vi "Event Handler.vi"(8 "error in (no error)":errorcluster, 10 "Stop Event Handler":refnum<user-event>, 11 "Cleaningcycle in":refnum<class "Cleaning cycle.lvclass">) -> (0 "error out":errorcluster)   [LabVIEW 2022 SP3, in "Cleaning cycle.lvclass"]
doc: "The <b>Event Handler VI</b> is a dynamic dispatch VI that should be overwritten if events are needed to create the enhanced QControl. \n\nBy inheriting from the main Control.lvclass the overwritten <b>Event Handler VI</b> will be launched asynchronously in the initialization of the QControl.\n<b> </b> <b> </b>\n©2016 Q Software Innovations, LLC (QSI)\nwritten by Quentin Alldredge\nproduced in LabVIEW 2015\n\nsupport@qsoftwareinnovations.com\nwww.qsoftwareinnovations.com\n\nAll rights reserved.\n\nRedistribution and use in source and binary forms, with or without modification, are permitted provided that the following conditions are met:\n\n * Redistributions of source code must retain the above copyright notice, this list of conditions and the following disclaimer.\n * Redistributions in binary form must reproduce the above copyright notice, this list of conditions and the following disclaimer in the documentation and/or other materials provided with the distribution.\n * Neither the name of Q Software Innovations, LLC. nor the names of its contributors may be used to endorse or promote products derived from this software without specific prior written permission.\n\nTHIS SOFTWARE IS PROVIDED BY THE COPYRIGHT HOLDERS AND CONTRIBUTORS \"AS IS\" AND ANY EXPRESS OR IMPLIED WARRANTIES, INCLUDING, BUT NOT LIMITED TO, THE IMPLIED WARRANTIES OF MERCHANTABILITY AND FITNESS FOR A PARTICULAR PURPOSE ARE DISCLAIMED. IN NO EVENT SHALL THE COPYRIGHT OWNER OR CONTRIBUTORS BE LIABLE FOR ANY DIRECT, INDIRECT, INCIDENTAL, SPECIAL, EXEMPLARY, OR CONSEQUENTIAL DAMAGES (INCLUDING, BUT NOT LIMITED TO, PROCUREMENT OF SUBSTITUTE GOODS OR SERVICES; LOSS OF USE, DATA, OR PROFITS; OR BUSINESS INTERRUPTION) HOWEVER CAUSED AND ON ANY THEORY OF LIABILITY, WHETHER IN CONTRACT, STRICT LIABILITY, OR TORT (INCLUDING NEGLIGENCE OR OTHERWISE) ARISING IN ANY WAY OUT OF THE USE OF THIS SOFTWARE, EVEN IF ADVISED OF THE POSSIBILITY OF SUCH DAMAGE."
uses:
  Cleaning cycle.lvclass
  Cleaning cycle.lvclass/Cleaning cycle.ctl
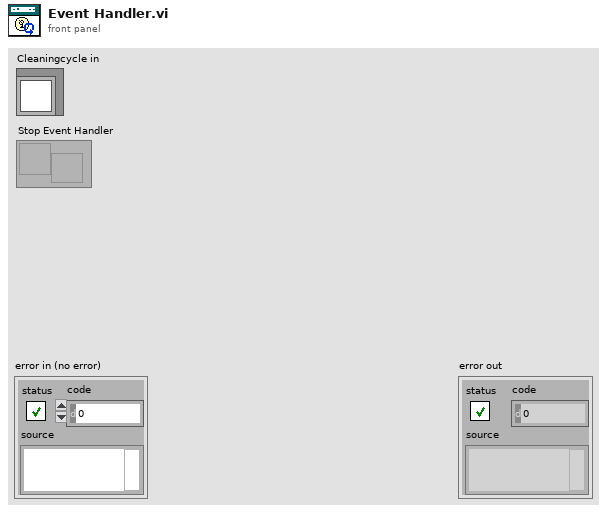
[diagram p1: front panel]
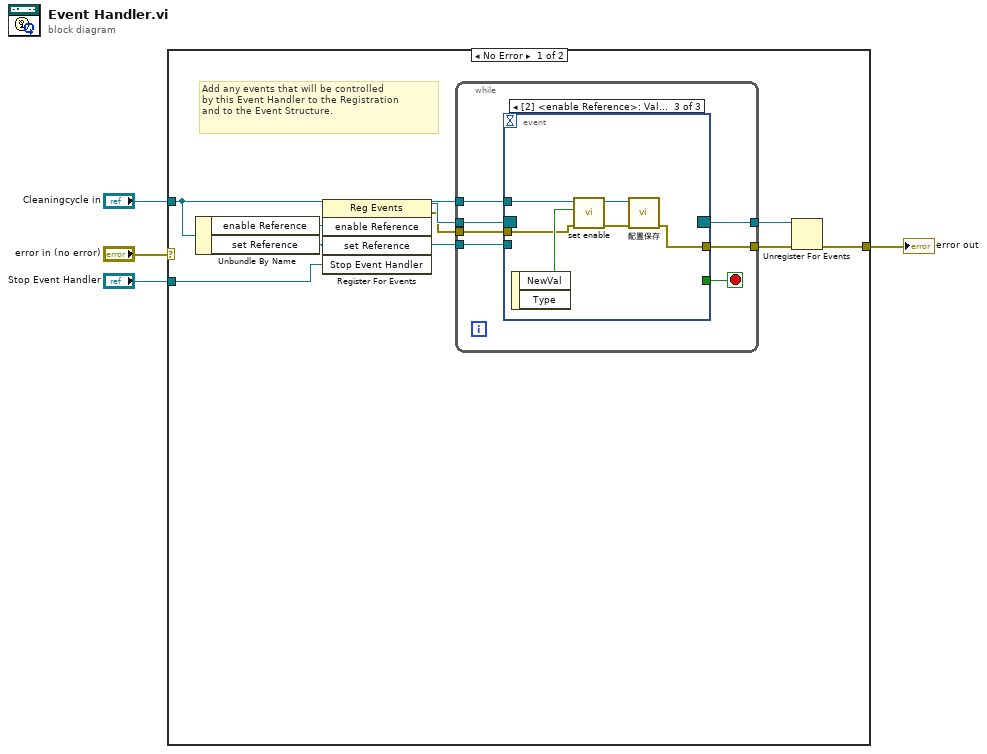
[diagram p0: block diagram]
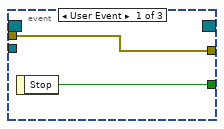
[diagram p2: hidden frame]
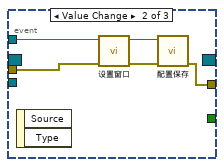
[diagram p3: hidden frame]
diagram:
  n1 = case shown="No Error" "error in (no error)" {
    selector: "error in (no error)" -> [_ w34]
    tunnel: [w11 w34] -> w3
    tunnel: "Cleaningcycle in" -> [w9 _]
    tunnel: "Stop Event Handler" -> [w5 _]
    frame No Error {
      # "Add any events that will be controlled\nby this Event Handler to the Registration\nand to the Event Structure."
      n2 = Unbundle By Name(w9) -> ("enable Reference"=w7:refnum<vi>, "set Reference"=w8:refnum<vi>)
      n3 = register-events(w7, w8, w5) -> (reference out=w13:refnum<event-registration>, error out=w6:errorcluster)  [unwired: 2 in]
      n4 = while {
        tunnel: w13 -> [w20]
        tunnel: w6 -> [w18]
        tunnel: [w17] -> w12
        tunnel: [w15] -> w10
        tunnel: w8 -> [w14]
        tunnel: w9 -> [w19]
        stop <- w16 stop-if-true
        n5 = event shown="[2] <enable Reference>: Value Change" {
          selector: w20 -> [_ _ _]
          dyn-events: [_ _ _] -> w15
          timeout: _ -> [_ _ _]
          tunnel: w19 -> [_ w27 w33]
          tunnel: w18 -> [w22 w24 w31]
          tunnel: [w22 w23 w28] -> w17
          tunnel: [w21 _ _] -> w16
          tunnel: w14 -> [_ _ _]
          event User Event {
            n6 = event-data() -> ("Stop"=w21:bool)  [unwired: 1 in]
          }
          event Value Change {
            n7 = event-data() -> ()  [unwired: 1 in, 2 out]
            n8 = call "设置窗口.vi"("error in (no error)"=w24, "Cleaningcycle in"=w27) -> ("error out"=w25:errorcluster, "Cleaningcycle out"=w26:refnum<class "Cleaning cycle.lvclass">)  [unwired: 8 in]
            n9 = call "配置保存.vi"("error in (no error)"=w25, "Cleaningcycle 输入"=w26) -> ("error out"=w23:errorcluster)  [unwired: 8 in, 1 out]
          }
          event Value Change {
            n10 = event-data() -> ("NewVal"=w32:bool)  [unwired: 1 in, 1 out]
            n11 = call "set enable.vi"("error in (no error)"=w31, "启用"=w32, "Cleaningcycle 输入"=w33) -> ("error out"=w29:errorcluster, "Cleaningcycle 输出"=w30:refnum<class "Cleaning cycle.lvclass">)  [unwired: 7 in]
            n12 = call "配置保存.vi"("error in (no error)"=w29, "Cleaningcycle 输入"=w30) -> ("error out"=w28:errorcluster)  [unwired: 8 in, 1 out]
          }
        }
      }
      n13 = Unregister For Events(event registration refnum=w10, error in=w12) -> (error out=w11:errorcluster)
    }
    frame Error {
    }
  }
  "error out" <- w3
